vi "insert.vi"(4 "footer (empty)":string[](array[string]), 5 "replace entry if exists (F)":bool, 6 "call chain index (1)":i32=1, 7 "vi ref (caller)":refnum<vi>, 8 "error in (no error)":errorcluster, 9 "body (empty)":string[](array[string]), 10 "header (empty)":string[](array[string]), 11 "summary control id":i32) -> (0 "error out":errorcluster)   [LabVIEW 2024, in "summary manager.lvlib"]
uses:
  summary manager.lvlib
  insert or remove.ctl
  entry type.ctl
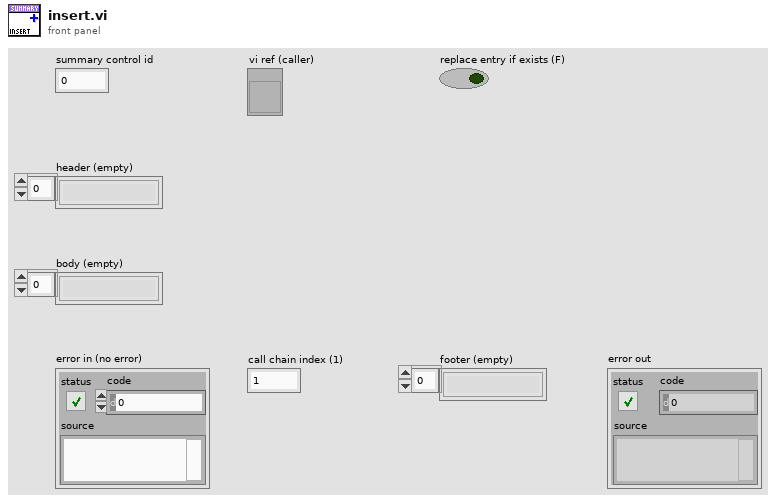
[diagram p1: front panel]
types:
  T1 = typedef "summary manager.lvlib/entry type.ctl" = cluster{"summary control id":i32, "header":string[], "body":string[], "footer":string[]}
  T2 = typedef "summary manager.lvlib/insert or remove.ctl" = enum16{"insert", "remove"}
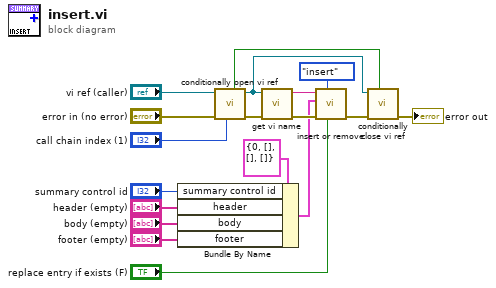
[diagram p0: block diagram]
diagram:
  n1 = Bundle By Name(cluster=T1 {"summary control id"=0, "header"=[], "body"=[], "footer"=[]}, "summary control id"="summary control id", "header"="header (empty)", "body"="body (empty)", "footer"="footer (empty)") -> (w5:T1)
  n2 = call "conditionally open vi ref.vi"("call chain index (1)"="call chain index (1)", "error in (no error)"="error in (no error)", "vi ref in"="vi ref (caller)") -> ("error out"=w16:errorcluster, "vi ref out"=w10:refnum<vi>, "new ref?"=w9:bool)  [unwired: 6 in]
  n3 = call "get vi name.vi"("error in (no error)"=w16, "vi ref"=w10) -> ("error out"=w14:errorcluster, "vi name"=w15:string)  [unwired: 8 in]
  n4 = call "insert or remove.vi"("replace entry if exists"="replace entry if exists (F)", "action"=insert_or_remove."insert", "error in (no error)"=w14, "entry"=w5, "id"=w15) -> ("error out"=w13:errorcluster)  [unwired: 6 in]
  n5 = call "conditionally close vi ref.vi"("new ref?"=w9, "error in (no error)"=w13, "vi ref"=w10) -> ("error out"=→"error out":errorcluster)  [unwired: 8 in]
